vi "create.volume.index.vi"(8 "error in (no error)":errorcluster, 9 "output filepath":path=path "D:/Comics/data/key_maps/volumes.json", 10 "Issue Path":path=path "D:/Comics/data/cv_issues", 11 "Volume Path":path=path "D:/Comics/data/cv_volumes") -> (0 "error out":errorcluster)   [LabVIEW 2024]
uses:
  definitions/volume.index--cluster.ctl
  volume.map--cluster.ctl
  definitions/volume.type--enum.ctl
  volume.index.content--cluster.ctl
  definitions/comicvine_issue.generic_credit.ctl
  <userlib>/_OpenG.lib/file/file.llb/Strip Path Extension - String__ogtk.vi
  <vilib>/addons/_JKI.lib/Serialization/JSON/JKI JSON Serialization.lvlib
  <userlib>/_OpenG.lib/file/file.llb/openg_file.lvlib
panel:
  out "current volume":string
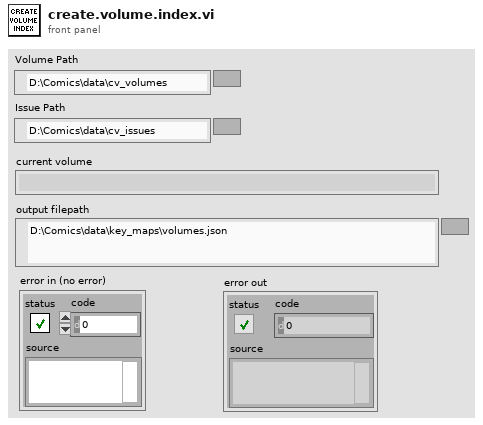
[diagram p1: front panel]
types:
  T1 = typedef "volume.map--cluster.ctl" = cluster{"volume":string, "characters":cluster{"id":i32, "name":string, "count":i32}[], "teams":cluster{"id":i32, "name":string, "count":i32}[], "start":timestamp, "end":timestamp, "count_of_issues":i32, "storyArcs":cluster{"id":i32, "name":string, "count":i32}[], "volume type":T2, "issues":cluster{"cover_date":timestamp, "id":i32, "number":string}[]}
  T2 = typedef "volume.type--enum.ctl" = enum16{"Ongoing", "Limited Series", "Annual", "One Shot", "Reprint/Document", "Star Comics", "Epic Comics"}
  T3 = typedef "volume.index.content--cluster.ctl" = cluster{"chars":map{T4, i32}, "teams":map{T4, i32}, "start":timestamp, "end":timestamp, "count_of_issues":i32, "storyArcs":map{T4, i32}, "volume type":T2, "issues":set{cluster{"id":i32, "number":string, "cover_date":timestamp}}}
  T4 = typedef "comicvine_issue.generic_credit.ctl" = cluster{"id":i32, "name":string}
  T5 = typedef "volume.index--cluster.ctl" = cluster{"volume_map":T1[]}
  T6 = typedef "local_volume.ctl" = cluster{"id":i32, "name":string, "sortable_name":string, "aliases":string[], "description":string, "site_detail_url":string, "count_of_issues":i32, "start_year":i32, "publisher_id":i32, "issue_ids":i32[], "date_last_updated":timestamp, "volume":i32, "cv_id":string, "volume type":T2}
  T7 = set{cluster{"id":i32, "number":string, "cover_date":timestamp}}
  T8 = typedef "local_issue.ctl" = cluster{"cover_date":timestamp, "id":i32, "cv_id":string, "name":string, "sortable_name":string, "issue_number":string, "deck":string, "description":string, "volume":T4, "store_date":timestamp, "date_last_updated":timestamp, "site_detail_url":string, "cover_url":string, "associated_images":T9[], "characters":T4[], "concepts":T4[], "creators":T10[], "storyArcs":T4[], "teams":T4[]}
  T9 = typedef "comicvine_issue.associated_image.ctl" = cluster{"original_url":string, "id":i32}
  T10 = typedef "comicvine_issue.person_credit.ctl" = cluster{"id":i32, "name":string, "role":string}
  T11 = cluster{"id":i32, "issue_number":string, "cover_date":timestamp}
  T12 = cluster{"cover_date":timestamp, "id":i32, "number":string}
  T13 = cluster{"cover_date":timestamp, "id":i32, "number":string}[]
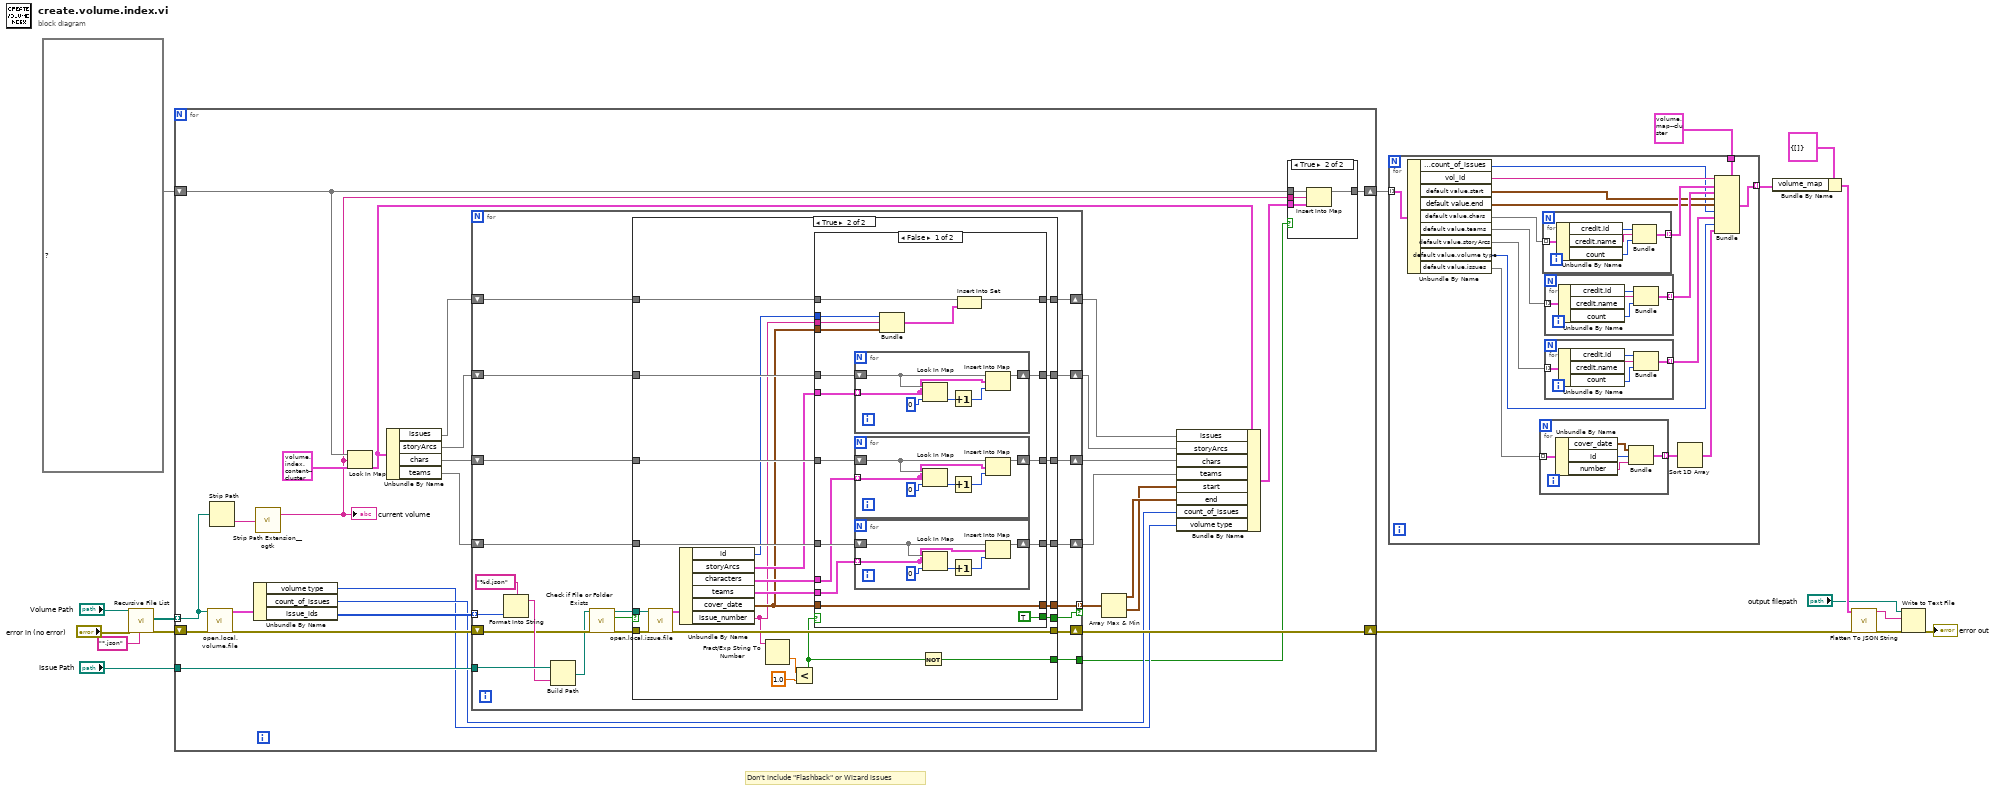
[diagram p0: block diagram]
diagram:
  # "Don't include \"Flashback\" or Wizard issues"
  n1 = call <vilib>:"Recursive File List.vi"("pattern"="*.json", "error in (no error)"="error in (no error)", "Folder Path"="Volume Path") -> ("error out"=w15:errorcluster, "All Files in Dir"=w14:path[])  [unwired: 4 in, 3 out]
  n2 = for {
    shift-right: [w39] -> w8
    shift-left: w15 -> [w45]
    tunnel: w14 -> [w38] mode=indexing
    tunnel: "Issue Path" -> [w42]
    shift-right: [w40] -> w12
    shift-left: map{string, T3} {} ("map") -> [w37]
    n3 = call "open.local.volume.file.vi"("error in (no error)"=w45, "volume json"=w38) -> ("error out"=w41:errorcluster, "volume"=w44:T6)  [unwired: 8 in]
    n4 = Strip Path(path=w38) -> (name=w21:string)  [unwired: 1 out]
    n5 = Unbundle By Name(w44) -> ("volume type"=w23:T2, "count_of_issues"=w26:i32, "issue_ids"=w43:i32[])
    n6 = call-poly <userlib>:"Strip Path Extension__ogtk.vi"("path"=w21) -> ("root"=w20:string)  [unwired: 1 out]
    "current volume" <- w20
    n7 = Look In Map(map=w37, key=w20, default value=T3 {"chars"={}, "teams"={}, "start"=timestamp(0 s since 1904-01-01), "end"=timestamp(0 s since 1904-01-01), "count_of_issues"=0, "storyArcs"={}, "volume type"=enum."Ongoing", "issues"={}}) -> (value=w33:T3)  [unwired: 1 out]
    n8 = Unbundle By Name(w33) -> ("issues"=w19:T7, "storyArcs"=w25:map{T4, i32}, "chars"=w34:map{T4, i32}, "teams"=w35:map{T4, i32})
    n9 = for {
      tunnel: w43 -> [w70] mode=indexing
      tunnel: w42 -> [w69]
      shift-right: [w60] -> w39
      shift-left: w41 -> [w67]
      shift-right: [w61] -> w31
      shift-left: w35 -> [w62]
      shift-right: [w58] -> w32
      shift-left: w34 -> [w59]
      tunnel: [w57] -> w29 mode=indexing if=w56
      shift-right: [w54] -> w24
      shift-left: w25 -> [w55]
      tunnel: [w53] -> w22
      shift-right: [w51] -> w18
      shift-left: w19 -> [w52]
      n10 = Format Into String(format string="%d.json", w70) -> (resulting string=w68:string)  [unwired: 2 in, 1 out]
      n11 = Build Path(base path=w69, name or relative path=w68) -> (appended path=w66:path)
      n12 = call <vilib>:"Check if File or Folder Exists.vi"("error in (no error)"=w67, "path"=w66) -> ("error out"=w63:errorcluster, "file or folder exists?"=w65:bool, "dup path"=w64:path)  [unwired: 7 in]
      n13 = case shown="True" w65 {
        tunnel: w64 -> [_ w100]
        tunnel: w63 -> [w75 w99]
        tunnel: w62 -> [w76 w97]
        tunnel: [w76 w96] -> w61
        tunnel: [w75 w95] -> w60
        tunnel: w59 -> [w74 w94]
        tunnel: [w74 w92] -> w58
        tunnel: [_ w89] -> w57
        tunnel: [_ w90] -> w56
        tunnel: w55 -> [w73 w85]
        tunnel: [w73 w84] -> w54
        tunnel: [_ w82] -> w53
        tunnel: w52 -> [w72 w81]
        tunnel: [w72 w77] -> w51
        frame False {
        }
        frame True {
          n14 = call "open.local.issue.file.vi"("error in (no error)"=w99, "volume json"=w100) -> ("error out"=w95:errorcluster, "issue"=w98:T8)  [unwired: 8 in]
          n15 = Unbundle By Name(w98) -> ("id"=w80:i32, "storyArcs"=w86:T4[], "characters"=w91:T4[], "teams"=w93:T4[], "cover_date"=w79:timestamp, "issue_number"=w78:string)
          n16 = Fract/Exp String To Number(string=w78) -> (number=w88:dbl)  [unwired: 3 in, 1 out]
          n17 = Less?(x=w88, y=1.0) -> (x < y?=w83:bool)
          n18 = case shown="False" w83 {
            tunnel: w97 -> [w117 w138]
            tunnel: [w116 w138] -> w96
            tunnel: w94 -> [w115 w139]
            tunnel: w93 -> [w114 _]
            tunnel: [w113 w139] -> w92
            tunnel: w91 -> [w112 _]
            tunnel: [TRUE _] -> w90
            tunnel: w79 -> [w110 _]
            tunnel: [w110 _] -> w89
            tunnel: w86 -> [w109 _]
            tunnel: w85 -> [w108 w137]
            tunnel: [w107 w137] -> w84
            tunnel: w81 -> [w103 w136]
            tunnel: w80 -> [w106 _]
            tunnel: w79 -> [w105 _]
            tunnel: w78 -> [w104 _]
            tunnel: [w101 w136] -> w77
            frame False {
              n19 = for {
                tunnel: w109 -> [w118] mode=indexing
                shift-right: [w119] -> w107
                shift-left: w108 -> [w120]
                n20 = Look In Map(map=w120, key=w118, default value=0) -> (value=w122:i32)  [unwired: 1 out]
                n21 = Increment(x=w122) -> (x+1=w121:i32)
                n22 = Insert Into Map(map in=w120, key=w118, value=w121) -> (map out=w119:map{T4, i32})  [unwired: 2 out]
              }
              n23 = for {
                tunnel: w112 -> [w124] mode=indexing
                shift-right: [w125] -> w113
                shift-left: w115 -> [w126]
                n24 = Look In Map(map=w126, key=w124, default value=0) -> (value=w128:i32)  [unwired: 1 out]
                n25 = Increment(x=w128) -> (x+1=w127:i32)
                n26 = Insert Into Map(map in=w126, key=w124, value=w127) -> (map out=w125:map{T4, i32})  [unwired: 2 out]
              }
              n27 = for {
                tunnel: w114 -> [w130] mode=indexing
                shift-right: [w131] -> w116
                shift-left: w117 -> [w132]
                n28 = Look In Map(map=w132, key=w130, default value=0) -> (value=w134:i32)  [unwired: 1 out]
                n29 = Increment(x=w134) -> (x+1=w133:i32)
                n30 = Insert Into Map(map in=w132, key=w130, value=w133) -> (map out=w131:map{T4, i32})  [unwired: 2 out]
              }
              n31 = Bundle("id"=w106, "issue_number"=w104, "cover_date"=w105) -> (w102:T11)  [unwired: 1 in]
              n32 = Insert Into Set(10:w102, 11:w103) -> (3:w101:T7)  [unwired: 1 out]
            }
            frame True {
            }
          }
          n33 = Not(x=w83) -> (.not. x?=w82:bool)
        }
      }
    }
    n34 = Array Max & Min(array=w29) -> (max value=w28:timestamp, min value=w27:timestamp)  [unwired: 2 out]
    n35 = Bundle By Name(cluster=w33, "issues"=w18, "storyArcs"=w24, "chars"=w32, "teams"=w31, "start"=w27, "end"=w28, "count_of_issues"=w26, "volume type"=w23) -> (w30:T3)
    n36 = case shown="True" w22 {
      tunnel: [w46 w50] -> w40
      tunnel: w37 -> [w46 w49]
      tunnel: w30 -> [_ w48]
      tunnel: w20 -> [_ w47]
      frame False {
      }
      frame True {
        n37 = Insert Into Map(map in=w49, key=w47, value=w48) -> (map out=w50:map{string, T3})  [unwired: 2 out]
      }
    }
  }
  n38 = for {
    tunnel: w12 -> [w156] mode=indexing
    tunnel: T1 {"volume"="", "characters"=[], "teams"=[], "start"=timestamp(0 s since 1904-01-01), "end"=timestamp(0 s since 1904-01-01), "count_of_issues"=0, "storyArcs"=[], "volume type"=enum."Ongoing", "issues"=[]} ("output cluster") -> [w154]
    tunnel: [w153] -> w10 mode=indexing
    n39 = Unbundle By Name(w156) -> ("default value.count_of_issues"=w146:i32, "vol_id"=w155:string, "default value.start"=w148:timestamp, "default value.end"=w147:timestamp, "default value.chars"=w149:map{T4, i32}, "default value.teams"=w152:map{T4, i32}, "default value.storyArcs"=w145:map{T4, i32}, "default value.volume type"=w143:T2, "default value.issues"=w142:T7)
    n40 = for {
      tunnel: w142 -> [w161] mode=indexing
      tunnel: [w158] -> w141 mode=indexing
      n41 = Unbundle By Name(w161) -> ("cover_date"=w157:timestamp, "id"=w160:i32, "number"=w159:string)
      n42 = Bundle("cover_date"=w157, "id"=w160, "number"=w159) -> (w158:T12)  [unwired: 1 in]
    }
    n43 = for {
      tunnel: w149 -> [w176] mode=indexing
      tunnel: [w173] -> w151 mode=indexing
      n44 = Unbundle By Name(w176) -> ("credit.id"=w175:i32, "credit.name"=w174:string, "count"=w172:i32)
      n45 = Bundle("id"=w175, "name"=w174, "count"=w172) -> (w173:cluster{"id":i32, "name":string, "count":i32})  [unwired: 1 in]
    }
    n46 = for {
      tunnel: w152 -> [w171] mode=indexing
      tunnel: [w168] -> w150 mode=indexing
      n47 = Unbundle By Name(w171) -> ("credit.id"=w170:i32, "credit.name"=w169:string, "count"=w167:i32)
      n48 = Bundle("id"=w170, "name"=w169, "count"=w167) -> (w168:cluster{"id":i32, "name":string, "count":i32})  [unwired: 1 in]
    }
    n49 = for {
      tunnel: w145 -> [w166] mode=indexing
      tunnel: [w163] -> w144 mode=indexing
      n50 = Unbundle By Name(w166) -> ("credit.id"=w165:i32, "credit.name"=w164:string, "count"=w162:i32)
      n51 = Bundle("id"=w165, "name"=w164, "count"=w162) -> (w163:cluster{"id":i32, "name":string, "count":i32})  [unwired: 1 in]
    }
    n52 = Sort 1D Array(array=w141) -> (sorted array=w140:T13)
    n53 = Bundle(cluster=w154, "volume"=w155, "characters"=w151, "teams"=w150, "start"=w148, "end"=w147, "count_of_issues"=w146, "storyArcs"=w144, "volume type"=w143, "issues"=w140) -> (w153:T1)
  }
  n54 = Bundle By Name(cluster=T5 {"volume_map"=[]}, "volume_map"=w10) -> (w9:T5)
  n55 = call <vilib>:"Flatten To JSON String.vi"("error in"=w8, "Variant"=w9) -> ("error out"=w7:errorcluster, "JSON String"=w6:string)  [unwired: 8 in]
  n56 = Write to Text File(file (use dialog)="output filepath", text=w6, error in=w7) -> (error out=→"error out":errorcluster)  [unwired: 1 in, 2 out]
